vi "LeerBD_externo.vi"(8 "error in (no error)":errorcluster) -> (0 "error out":errorcluster, 2 "BD":T1={"frec_referencia"=98.0, "niv_presion_son_ref"=97.0, "Incertidumbre"=["1", "1", "1", "1", "1", "1", "1", "1", "1", "1"], "Tol +"=["2,0", "1,5", "1,5", "1,4", "1,4", "1,1", "1,6", "1,6", "2,1", "3,5"], "Tol -"=["-2,0", "-1,5", "-1,5", "-1,4", "-1,4", "-1,1", "-1,6", "-1,6", "-2,1", "-3,5"], "Referencia(dB)"=["95", "94", "94", "94", "96", "95", "94", "96", "95", "94"], "Frecuencias(Hz)"=["95", "94", "94", "94", "96", "95", "94", "96", "95", "94"], "vol_enviado_CAM"=0.0, "CorreccionMic"=["95", "94", "94", "94", "96", "95", "94", "96", "95", "94"]}, 3 "Prueba02 out":refnum<class "Prueba02.lvclass">)   [LabVIEW 2019, in "Prueba03.lvclass"]
uses:
  Prueba03.lvclass
  Prueba02/Prueba02.lvclass
  Controles/BD.ctl
  Base de Datos/SQLiteConnector/SQLiteConnection.lvclass
  Base de Datos/Base de Datos.lvclass
panel:
  in  "Tipo Equipo":enum16{"Sonometro", "Calibrador", "Dosimetro"}(ring)
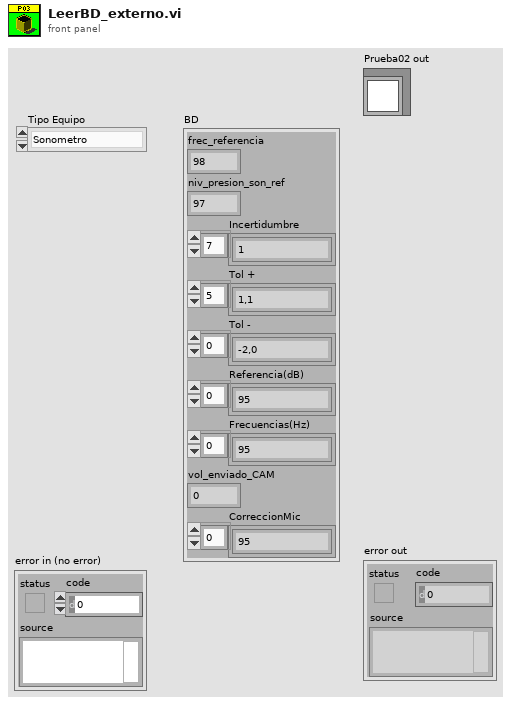
[diagram p1: front panel]
types:
  T1 = typedef "Prueba03.lvclass/BD.ctl" = cluster{"frec_referencia":dbl, "niv_presion_son_ref":dbl, "Incertidumbre":string[], "Tol +":string[], "Tol -":string[], "Referencia(dB)":string[], "Frecuencias(Hz)":string[], "vol_enviado_CAM":dbl, "CorreccionMic":string[]}
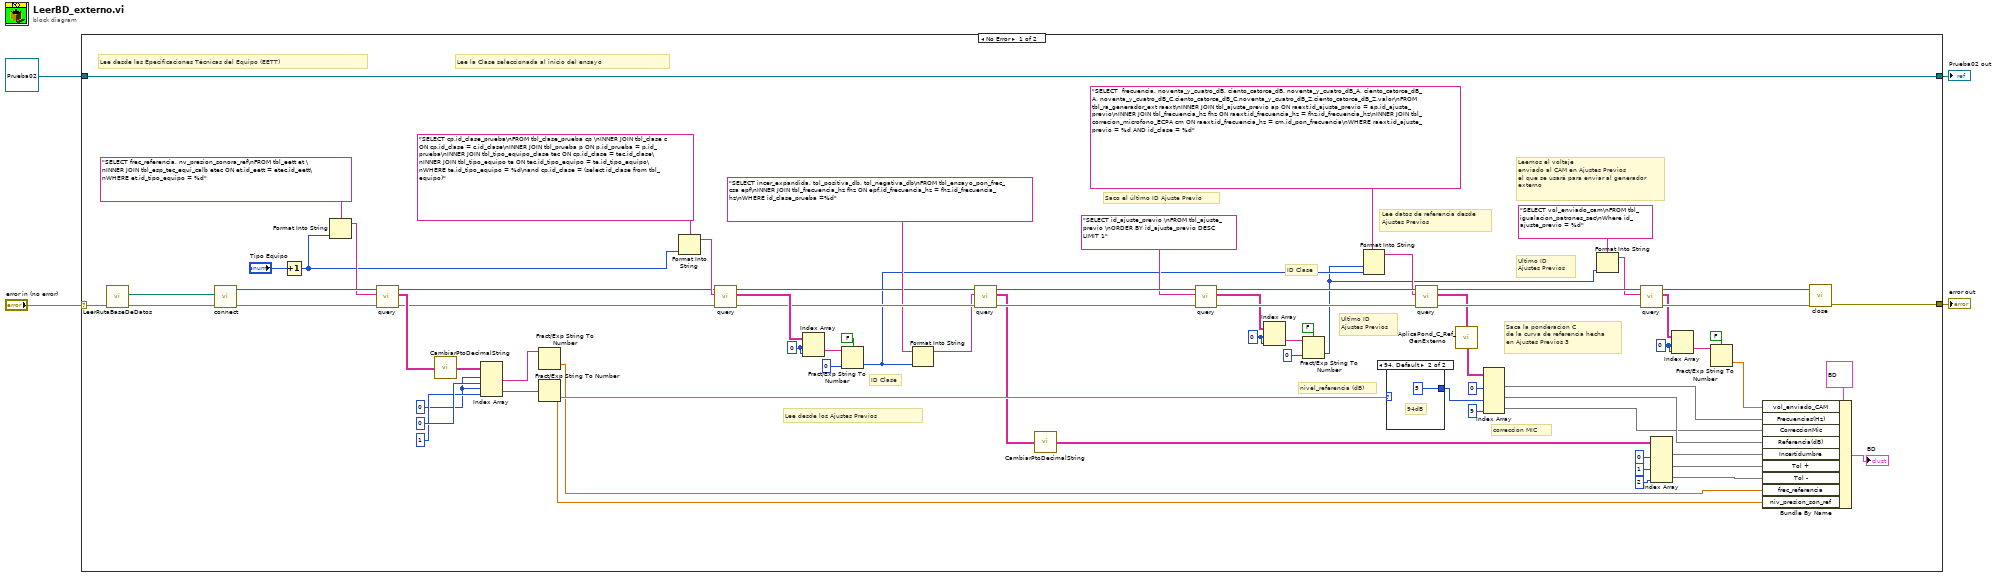
[diagram p0: block diagram]
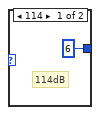
[diagram p2: hidden frame]
diagram:
  n1 = case shown="No Error" "error in (no error)" {
    selector: "error in (no error)" -> [w72 w84]
    tunnel: [w56 w84] -> w3
    tunnel: [w80 w83] -> w1
    tunnel: refnum<class "Prueba02.lvclass"> refnum ("Prueba02 in") -> [w80 w83]
    frame No Error {
      w16 = 0 ("index (row)")
      w30 = 0 ("index (row)")
      w62 = 0 ("index (row)")
      w55 = 0 ("index (row)")
      # "correccion MIC"
      # "Saca la ponderacion C\nde la curva de referencia hecha\nen Ajustes Previos 3"
      # "Ultimo ID\nAjustes Previos"
      # "Ultimo ID\nAjustes Previos"
      # "ID Clase"
      # "Leemos el voltaje\nenviado al CAM en Ajustes Previos\nel que se usará para enviar al generador\nexterno"
      # "Lee datos de referencia desde\nAjustes Previos"
      # "ID Clase"
      # "Saco el último ID Ajuste Previo"
      # "nivel_referencia (dB)"
      # "Lee desde los Ajustes Previos"
      # "Lee la Clase seleccionada al inicio del ensayo"
      # "Lee desde las Epecificaciones Técnicas del Equipo (EETT)"
      n2 = call "LeerRutaBaseDeDatos.vi"("error in (no error)"=w72) -> ("error out"=w75:errorcluster, "Database Path"=w74:path)  [unwired: 9 in]
      n3 = call "connect.vi"("error in (no error)"=w75, "Database Path"=w74) -> ("error out"=w77:errorcluster, "object out"=w78:refnum<class "SQLiteConnection.lvclass">)  [unwired: 8 in]
      n4 = Increment(x="Tipo Equipo") -> (x+1=w49:enum16{"Sonometro", "Calibrador", "Dosimetro"})
      n5 = Format Into String(format string="SELECT frec_referencia, nv_presion_sonora_ref\nFROM tbl_eett et \nINNER JOIN tbl_esp_tec_equi_calb etec ON et.id_eett = etec.id_eett\nWHERE et.id_tipo_equipo = %d", w49) -> (resulting string=w76:string)  [unwired: 2 in, 1 out]
      n6 = call "query.vi"("error in (no error)"=w77, "SQL Statement"=w76, "object in"=w78) -> ("error out"=w63:errorcluster, "result"=w67:string[][], "object out"=w64:refnum<class "SQLiteConnection.lvclass">)  [unwired: 5 in, 1 out]
      n7 = call "CambiarPtoDecimalString.vi"("result"=w67) -> ("result out"=w9:string[][])
      n8 = Index Array(array=w9, index (row) #1=w55, index (col) #1=0 ("disabled index (col)"), index (row) #2=w55, index (col) #2=1 ("disabled index (col)")) -> (element #1=w69:string, element #2=w68:string)
      n9 = Fract/Exp String To Number(string=w69) -> (number=w38:dbl)  [unwired: 3 in, 1 out]
      n10 = Fract/Exp String To Number(string=w68) -> (number=w48:dbl)  [unwired: 3 in, 1 out]
      n11 = Format Into String(format string="SELECT cp.id_clase_prueba\nFROM tbl_clase_prueba cp \nINNER JOIN tbl_clase c ON cp.id_clase = c.id_clase\nINNER JOIN tbl_prueba p ON p.id_prueba = p.id_prueba\nINNER JOIN tbl_tipo_equipo_clase tec ON cp.id_clase = tec.id_clase\nINNER JOIN tbl_tipo_equipo te ON tec.id_tipo_equipo = te.id_tipo_equipo\nWHERE te.id_tipo_equipo = %d\nand cp.id_clase = (select id_clase from tbl_equipo)", w49) -> (resulting string=w65:string)  [unwired: 2 in, 1 out]
      n12 = call "query.vi"("error in (no error)"=w63, "SQL Statement"=w65, "object in"=w64) -> ("error out"=w57:errorcluster, "result"=w58:string[][], "object out"=w52:refnum<class "SQLiteConnection.lvclass">)  [unwired: 5 in, 1 out]
      n13 = Index Array(array=w58, index (row)=w62, index (col)=w62) -> (element=w60:string)
      n14 = Fract/Exp String To Number(use system decimal point (T)=FALSE, string=w60, default (0 dbl)=0 ("index (row)")) -> (number=w26:i32)  [unwired: 1 in, 1 out]
      n15 = Format Into String(format string="SELECT incer_expandida, tol_positiva_db, tol_negativa_db\nFROM tbl_ensayo_pon_frec_csa epf\nINNER JOIN tbl_frecuencia_hz fhz ON epf.id_frecuencia_hz = fhz.id_frecuencia_hz\nWHERE id_clase_prueba =%d", w26) -> (resulting string=w51:string)  [unwired: 2 in, 1 out]
      n16 = call "query.vi"("error in (no error)"=w57, "SQL Statement"=w51, "object in"=w52) -> ("error out"=w53:errorcluster, "result"=w43:string[][], "object out"=w36:refnum<class "SQLiteConnection.lvclass">)  [unwired: 5 in, 1 out]
      n17 = call "CambiarPtoDecimalString.vi"("result"=w43) -> ("result out"=w10:string[][])
      n18 = call "query.vi"("error in (no error)"=w53, "SQL Statement"="SELECT id_ajuste_previo \nFROM tbl_ajuste_previo \nORDER BY id_ajuste_previo DESC LIMIT 1" ("format string"), "object in"=w36) -> ("error out"=w37:errorcluster, "result"=w29:string[][], "object out"=w35:refnum<class "SQLiteConnection.lvclass">)  [unwired: 5 in, 1 out]
      n19 = Index Array(array=w29, index (row)=w30, index (col)=w30) -> (element=w32:string)
      n20 = Fract/Exp String To Number(use system decimal point (T)=FALSE, string=w32, default (0 dbl)=0 ("index (row)")) -> (number=w19:i32)  [unwired: 1 in, 1 out]
      n21 = Format Into String(format string="SELECT  frecuencia, noventa_y_cuatro_dB, ciento_catorce_dB, noventa_y_cuatro_dB_A, ciento_catorce_dB_A, noventa_y_cuatro_dB_C,ciento_catorce_dB_C,noventa_y_cuatro_dB_Z,ciento_catorce_dB_Z,valor\nFROM tbl_ra_generador_ext raext\nINNER JOIN tbl_ajuste_previo ap ON raext.id_ajuste_previo = ap.id_ajuste_previo\nINNER JOIN tbl_frecuencia_hz fhz ON raext.id_frecuencia_hz = fhz.id_frecuencia_hz\nINNER JOIN tbl_correcion_microfono_ECPA cm ON raext.id_frecuencia_hz = cm.id_pon_frecuencia\nWHERE raext.id_ajuste_previo = %d AND id_clase = %d", w19, w26) -> (resulting string=w27:string)  [unwired: 2 in, 1 out]
      n22 = case shown="94, Default" w48 {
        tunnel: [6 ("disabled index (col)") 5 ("disabled index (col)")] -> w13
        frame 114 {
          # "114dB"
        }
        frame 94, Default {
          # "94dB"
        }
      }
      n23 = call "query.vi"("error in (no error)"=w37, "SQL Statement"=w27, "object in"=w35) -> ("error out"=w50:errorcluster, "result"=w12:string[][], "object out"=w23:refnum<class "SQLiteConnection.lvclass">)  [unwired: 5 in, 1 out]
      n24 = call "AplicaPond_C_Ref_GenExterno.vi"("result"=w12) -> ("output array"=w11:string[][])
      n25 = Index Array(array=w11, index (col) #1=0 ("disabled index (col)"), index (col) #2=w13, index (col) #3=9 ("index (col)")) -> (element #1=w7:string[], element #2=w14:string[], element #3=w5:string[])  [unwired: 3 in]
      n26 = Format Into String(format string="SELECT vol_enviado_cam\nFROM tbl_igualacion_patrones_sec\nWhere id_ajuste_previo = %d", w19) -> (resulting string=w20:string)  [unwired: 2 in, 1 out]
      n27 = call "query.vi"("error in (no error)"=w50, "SQL Statement"=w20, "object in"=w23) -> ("error out"=w24:errorcluster, "result"=w15:string[][], "object out"=w22:refnum<class "SQLiteConnection.lvclass">)  [unwired: 5 in, 1 out]
      n28 = Index Array(array=w10, index (col) #1=0 ("disabled index (col)"), index (col) #2=1 ("index (col)"), index (col) #3=2 ("index (col)")) -> (element #1=w46:string[], element #2=w45:string[], element #3=w44:string[])  [unwired: 3 in]
      n29 = Index Array(array=w15, index (row)=w16, index (col)=w16) -> (element=w18:string)
      n30 = Fract/Exp String To Number(use system decimal point (T)=FALSE, string=w18) -> (number=w8:dbl)  [unwired: 2 in, 1 out]
      n31 = Bundle By Name(cluster=T1 {"frec_referencia"=98.0, "niv_presion_son_ref"=97.0, "Incertidumbre"=["1", "1", "1", "1", "1", "1", "1", "1", "1", "1"], "Tol +"=["2,0", "1,5", "1,5", "1,4", "1,4", "1,1", "1,6", "1,6", "2,1", "3,5"], "Tol -"=["-2,0", "-1,5", "-1,5", "-1,4", "-1,4", "-1,1", "-1,6", "-1,6", "-2,1", "-3,5"], "Referencia(dB)"=["95", "94", "94", "94", "96", "95", "94", "96", "95", "94"], "Frecuencias(Hz)"=["95", "94", "94", "94", "96", "95", "94", "96", "95", "94"], "vol_enviado_CAM"=0.0, "CorreccionMic"=["95", "94", "94", "94", "96", "95", "94", "96", "95", "94"]} ("BD"), "vol_enviado_CAM"=w8, "Frecuencias(Hz)"=w7, "CorreccionMic"=w5, "Referencia(dB)"=w14, "Incertidumbre"=w46, "Tol +"=w45, "Tol -"=w44, "frec_referencia"=w38, "niv_presion_son_ref"=w48) -> (→"BD":T1)
      n32 = call-dynamic "close.vi"("error in (no error)"=w24, "object in"=w22) -> ("error out"=w56:errorcluster)  [unwired: 8 in, 1 out]
    }
    frame Error {
    }
  }
  "error out" <- w3
  "Prueba02 out" <- w1
